vi "Variant to array strings.vi"(5 "cluster":T2(array[cluster]), 6 "Array index":string, 8 "Error out":errorcluster, 9 "Path":string, 10 "Params":T3, 11 "Variant":variant) -> (0 "Error out":errorcluster, 3 "output array":T2(array[cluster]))   [LabVIEW 2021, in "Tree.lvlib" / "Tree.lvclass"]
uses:
  Tree.lvclass
  <vilib>/Utility/Data Type/Type Definitions/Data Type.ctl
  <vilib>/Utility/Data Type/NI_Data Type.lvlib
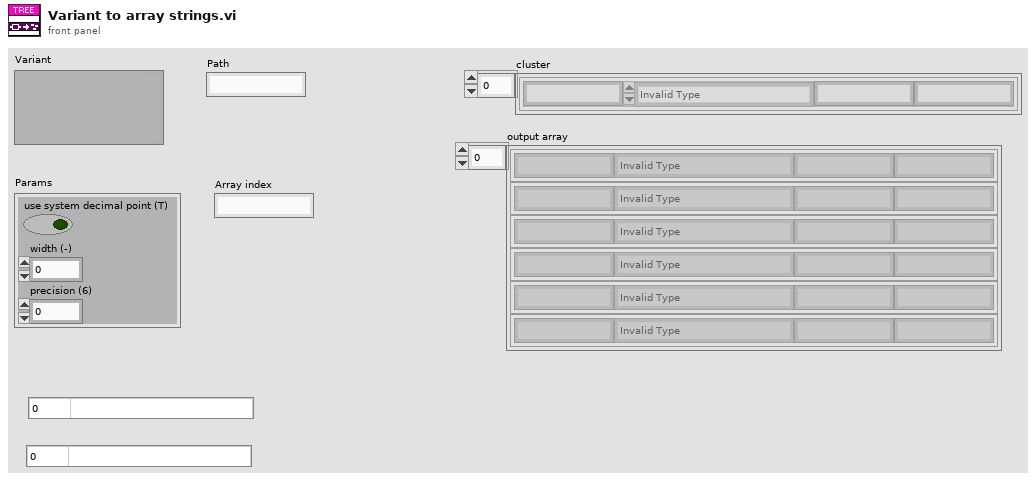
[diagram p1: front panel]
types:
  T1 = typedef "NI_Data Type.lvlib/Data Type.ctl" = enum8{"Invalid Type", "Void", "I8", "I16", "I32", "I64", "U8", "U16", "U32", "U64", "Single Float", "Double Float", "Extended Float", "Single Complex", "Double Complex", "Extended Complex", "Enum U8", "Enum U16", "Enum U32", "Enum U64", "Single Float With Unit", "Double Float With Unit", "Extended Float With Unit", "Single Complex with Unit", "Double Complex with Unit", "Extended Complex with Unit", "Boolean", "String", "Path", "Picture", "Tag", "Array", "Cluster", "Variant", "LV Variant", "Waveform", "Timestamp", "Digital Waveform", "Digital Data", "ExpressData", "Refnum", "External Data", "VI", "Poly VI", "LabVIEW Class Instance", "Fixed Point", "Set Collection", "Map Collection"}
  T2 = cluster{"Path":string, "Type":T1, "Label":string, "Value":string}[]
  T3 = cluster{"use system decimal point (T)":bool, "width (-)":i16, "precision (6)":i16}
  T4 = cluster{"Path":string, "type":T1, string, string}
  T5 = cluster{"Path":string, "type":T1, "Label":string, "Value":string}[]
  T6 = cluster{"Path":string, "type":T1, string, "Name":string}
  T7 = cluster{"Path":string, "type":T1, "Label":string, "Name":string}[]
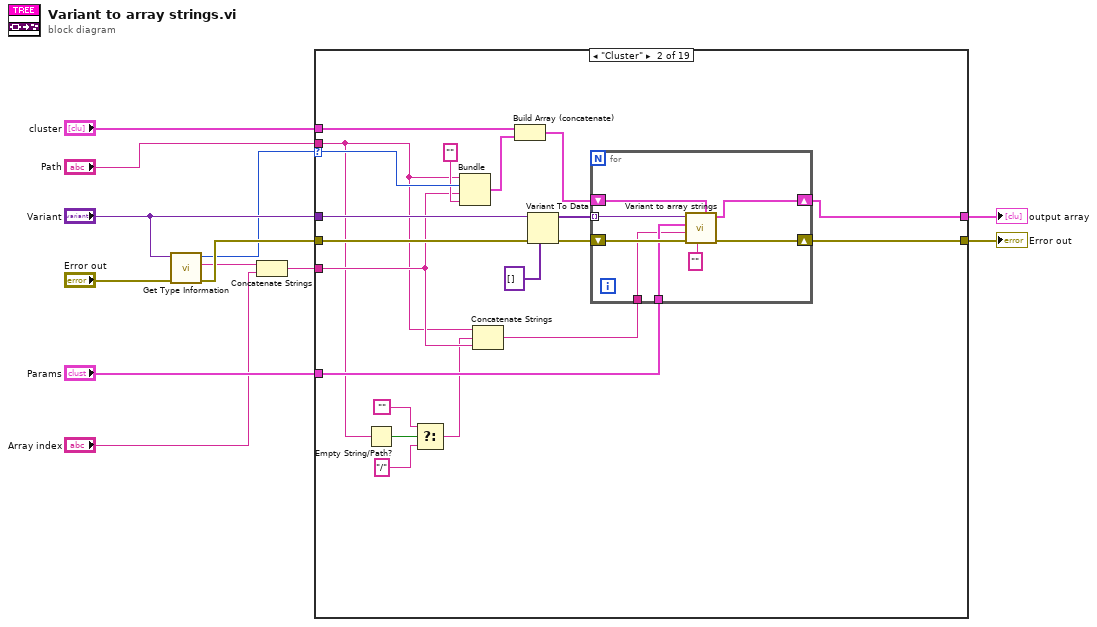
[diagram p0: block diagram]
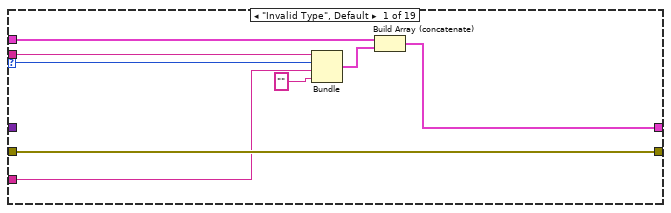
[diagram p2: hidden frame]
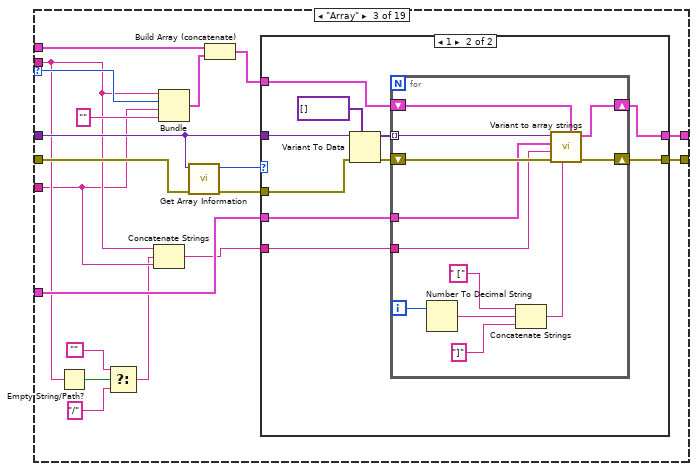
[diagram p3: hidden frame]
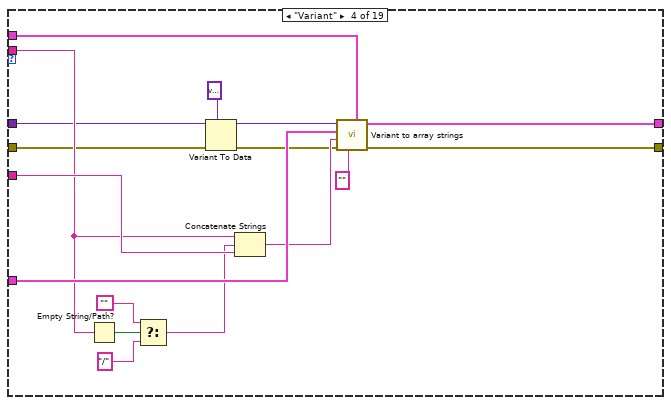
[diagram p5: hidden frame]
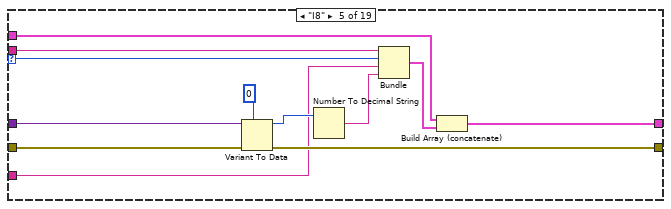
[diagram p6: hidden frame]
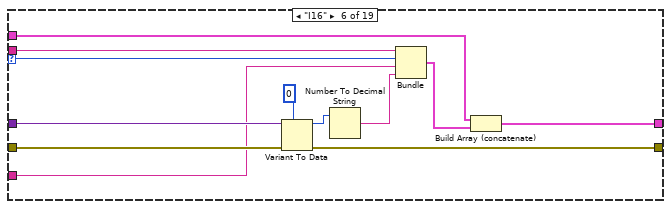
[diagram p7: hidden frame]
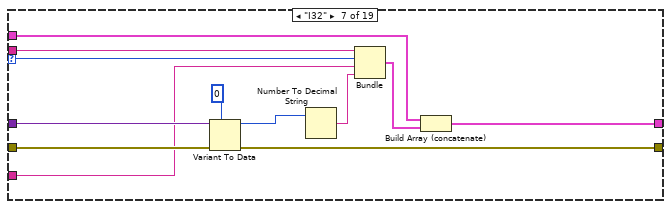
[diagram p8: hidden frame]
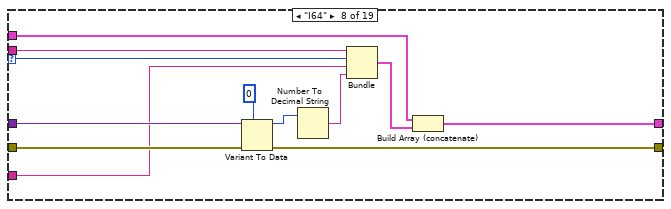
[diagram p9: hidden frame]
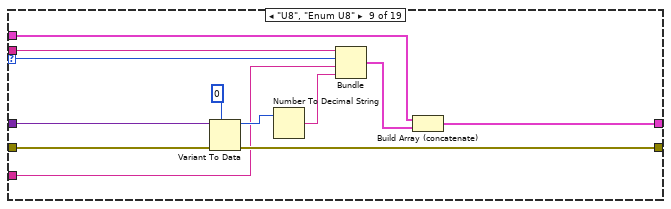
[diagram p10: hidden frame]
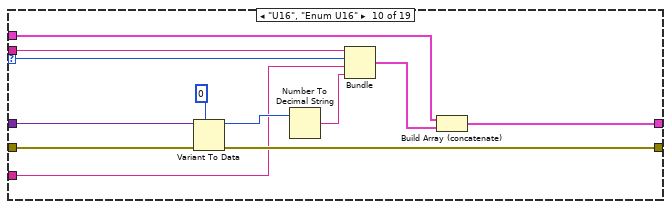
[diagram p11: hidden frame]
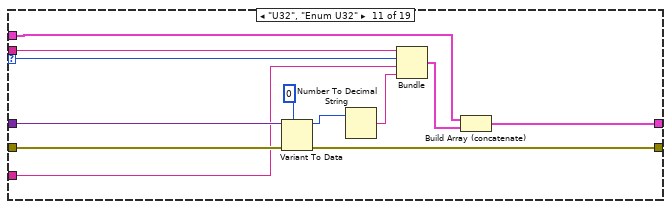
[diagram p12: hidden frame]
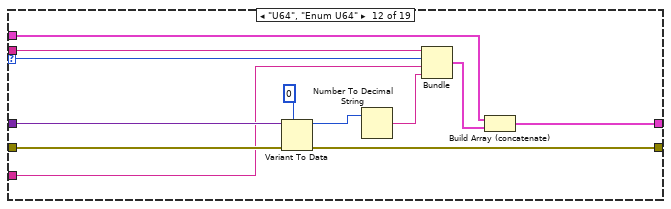
[diagram p13: hidden frame]
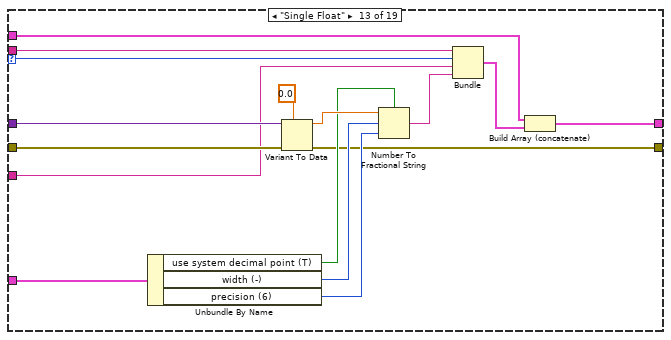
[diagram p14: hidden frame]
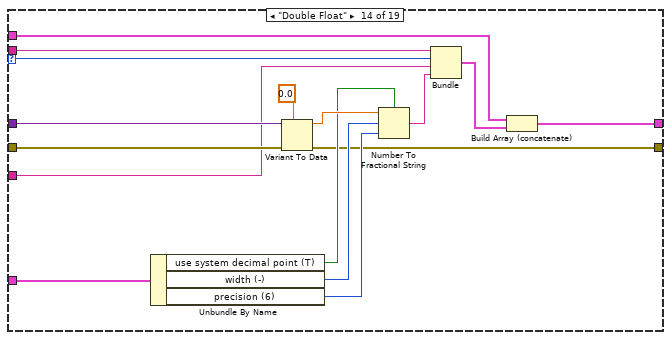
[diagram p15: hidden frame]
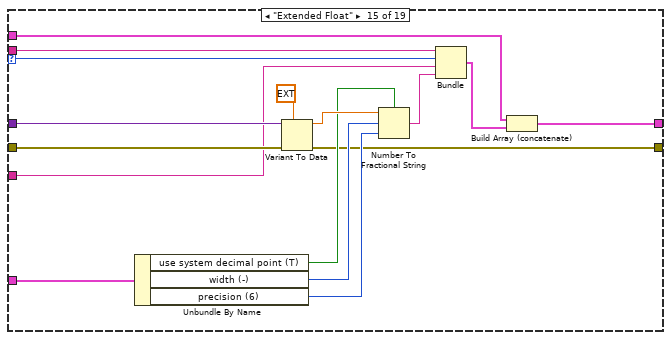
[diagram p16: hidden frame]
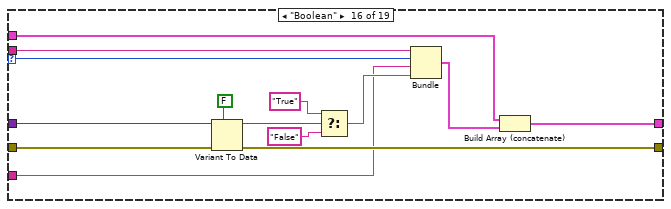
[diagram p17: hidden frame]
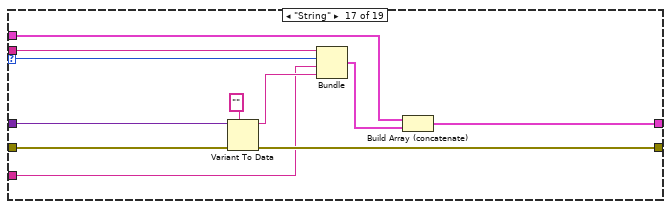
[diagram p18: hidden frame]
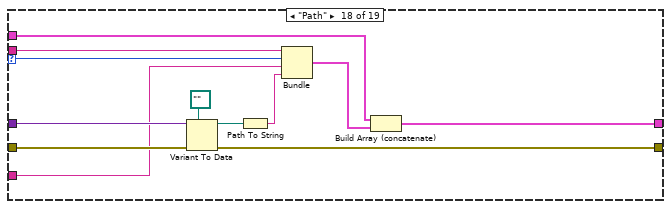
[diagram p19: hidden frame]
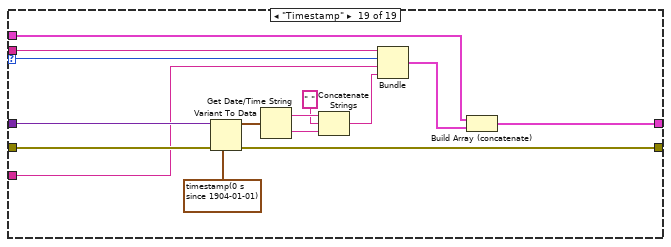
[diagram p20: hidden frame]
diagram:
  n1 = call <vilib>:"Get Type Information.vi"("error in (no error)"="Error out", "variant"="Variant") -> ("error out"=w11:errorcluster, "name"=w7:string, "type"=w9:T1)  [unwired: 5 in, 2 out]
  n2 = Concatenate Strings(w7, "Array index") -> (w2:string)
  n3 = case shown="\"Cluster\"" w9 {
    selector: w9 -> [w19 w36 w59 _ w114 w126 w138 w150 w162 w174 w186 w198 w205 w226 w242 w258 w272 w281 w295]
    tunnel: "Variant" -> [_ w33 w64 w97 w120 w132 w144 w156 w168 w180 w192 w204 w220 w236 w252 w266 w277 w289 w304]
    tunnel: w11 -> [w20 w31 w62 w94 w116 w128 w140 w152 w164 w176 w188 w200 w212 w228 w244 w264 w276 w288 w303]
    tunnel: [w20 w40 w65 w108 w115 w127 w139 w151 w163 w175 w187 w199 w211 w227 w243 w263 w275 w287 w302] -> w8
    tunnel: w2 -> [w13 w26 w50 w103 w109 w121 w133 w145 w157 w169 w181 w193 w206 w221 w237 w253 w267 w278 w290]
    tunnel: [w16 w38 w66 w106 w117 w129 w141 w153 w165 w177 w189 w201 w218 w234 w250 w260 w274 w286 w301] -> w5
    tunnel: "Params" -> [_ w39 w67 w107 _ _ _ _ _ _ _ _ w216 w232 w248 _ _ _ _]
    tunnel: "cluster" -> [w15 w37 w60 w105 w111 w123 w135 w147 w159 w171 w183 w195 w208 w223 w239 w255 w270 w280 w292]
    tunnel: "Path" -> [w14 w25 w51 w99 w110 w122 w134 w146 w158 w170 w182 w194 w207 w222 w238 w254 w268 w279 w291]
    frame "Invalid Type", Default {
      n4 = Bundle("Path"=w14, "type"=w19, w13, "") -> (w17:T4)  [unwired: 1 in]
      n5 = Build Array (concatenate)(w15, w17) -> (w16:T5)
    }
    frame "Cluster" {
      n6 = Empty String/Path?(string/path=w25) -> (empty?=w24:bool)
      n7 = Select(t="", s=w24, f="/" ("string")) -> (s? t:f=w21:string)
      n8 = Bundle("Path"=w25, "type"=w36, w26, "") -> (w27:T4)  [unwired: 1 in]
      n9 = Concatenate Strings(w25, w21, w26) -> (w35:string)
      n10 = Build Array (concatenate)(w37, w27) -> (w28:T5)
      n11 = Variant To Data(error in=w31, type=variant[] [], Variant=w33) -> (data=w29:variant[], error out=w30:errorcluster)
      n12 = for {
        shift-right: [w47] -> w40
        shift-left: w30 -> [w48]
        tunnel: w29 -> [w46] mode=indexing
        tunnel: w39 -> [w45]
        shift-right: [w42] -> w38
        shift-left: w28 -> [w44]
        tunnel: w35 -> [w43]
        n13 = call "Variant to array strings.vi"("cluster"=w44, "Array index"="", "Error out"=w48, "Path"=w43, "Params"=w45, "Variant"=w46) -> ("Error out"=w47:errorcluster, "output array"=w42:T2)  [unwired: 4 in]
      }
    }
    frame "Array" {
      n14 = Empty String/Path?(string/path=w51) -> (empty?=w54:bool)
      n15 = Select(t="", s=w54, f="/" ("string")) -> (s? t:f=w49:string)
      n16 = Concatenate Strings(w51, w49, w50) -> (w58:string)
      n17 = Bundle("Path"=w51, "type"=w59, w50, "") -> (w55:T4)  [unwired: 1 in]
      n18 = call <vilib>:"Get Array Information.vi"("error in (no error)"=w62, "variant"=w64) -> ("error out"=w61:errorcluster, "number of dimensions"=w63:i32)  [unwired: 6 in, 2 out]
      n19 = Build Array (concatenate)(w60, w55) -> (w56:T5)
      n20 = case shown="1" w63 {
        tunnel: w67 -> [_ w79]
        tunnel: [w68 w78] -> w66
        tunnel: [w69 w77] -> w65
        tunnel: w64 -> [_ w74]
        tunnel: w61 -> [w69 w73]
        tunnel: w56 -> [w68 w71]
        tunnel: w58 -> [_ w70]
        frame 0, Default {
        }
        frame 1 {
          n21 = Variant To Data(error in=w73, type=variant[] [], Variant=w74) -> (data=w75:variant[], error out=w72:errorcluster)
          n22 = for {
            tunnel: w75 -> [w91] mode=indexing
            shift-right: [w89] -> w77
            shift-left: w72 -> [w90]
            tunnel: w79 -> [w88]
            shift-right: [w87] -> w78
            shift-left: w71 -> [w86]
            tunnel: w70 -> [w85]
            i -> [w84]
            n23 = Number To Decimal String(number=w84) -> (decimal integer string=w83:string)  [unwired: 1 in]
            n24 = Concatenate Strings(" [" ("string"), w83, "]" ("string")) -> (w80:string)
            n25 = call "Variant to array strings.vi"("cluster"=w86, "Array index"=w80, "Error out"=w90, "Path"=w85, "Params"=w88, "Variant"=w91) -> ("Error out"=w89:errorcluster, "output array"=w87:T2)  [unwired: 4 in]
          }
        }
      }
    }
    frame "Variant" {
      n26 = Empty String/Path?(string/path=w99) -> (empty?=w102:bool)
      n27 = Select(t="", s=w102, f="/" ("string")) -> (s? t:f=w98:string)
      n28 = Variant To Data(error in=w94, type=variant, Variant=w97) -> (data=w95:variant, error out=w93:errorcluster)
      n29 = Concatenate Strings(w99, w98, w103) -> (w104:string)
      n30 = call "Variant to array strings.vi"("cluster"=w105, "Array index"="", "Error out"=w93, "Path"=w104, "Params"=w107, "Variant"=w95) -> ("Error out"=w108:errorcluster, "output array"=w106:T2)  [unwired: 4 in]
    }
    frame "I8" {
      n31 = Variant To Data(error in=w116, type=i8 0, Variant=w120) -> (data=w118:i8, error out=w115:errorcluster)
      n32 = Number To Decimal String(number=w118) -> (decimal integer string=w113:string)  [unwired: 1 in]
      n33 = Bundle("Path"=w110, "type"=w114, w109, w113) -> (w112:T4)  [unwired: 1 in]
      n34 = Build Array (concatenate)(w111, w112) -> (w117:T5)
    }
    frame "I16" {
      n35 = Variant To Data(error in=w128, type=i16 0, Variant=w132) -> (data=w130:i16, error out=w127:errorcluster)
      n36 = Number To Decimal String(number=w130) -> (decimal integer string=w125:string)  [unwired: 1 in]
      n37 = Bundle("Path"=w122, "type"=w126, w121, w125) -> (w124:T4)  [unwired: 1 in]
      n38 = Build Array (concatenate)(w123, w124) -> (w129:T5)
    }
    frame "I32" {
      n39 = Variant To Data(error in=w140, type=0, Variant=w144) -> (data=w142:i32, error out=w139:errorcluster)
      n40 = Number To Decimal String(number=w142) -> (decimal integer string=w137:string)  [unwired: 1 in]
      n41 = Bundle("Path"=w134, "type"=w138, w133, w137) -> (w136:T4)  [unwired: 1 in]
      n42 = Build Array (concatenate)(w135, w136) -> (w141:T5)
    }
    frame "I64" {
      n43 = Variant To Data(error in=w152, type=i64 0, Variant=w156) -> (data=w154:i64, error out=w151:errorcluster)
      n44 = Number To Decimal String(number=w154) -> (decimal integer string=w149:string)  [unwired: 1 in]
      n45 = Bundle("Path"=w146, "type"=w150, w145, w149) -> (w148:T4)  [unwired: 1 in]
      n46 = Build Array (concatenate)(w147, w148) -> (w153:T5)
    }
    frame "U8", "Enum U8" {
      n47 = Variant To Data(error in=w164, type=u8 0, Variant=w168) -> (data=w166:u8, error out=w163:errorcluster)
      n48 = Number To Decimal String(number=w166) -> (decimal integer string=w161:string)  [unwired: 1 in]
      n49 = Bundle("Path"=w158, "type"=w162, w157, w161) -> (w160:T4)  [unwired: 1 in]
      n50 = Build Array (concatenate)(w159, w160) -> (w165:T5)
    }
    frame "U16", "Enum U16" {
      n51 = Variant To Data(error in=w176, type=u16 0, Variant=w180) -> (data=w178:u16, error out=w175:errorcluster)
      n52 = Number To Decimal String(number=w178) -> (decimal integer string=w173:string)  [unwired: 1 in]
      n53 = Bundle("Path"=w170, "type"=w174, w169, w173) -> (w172:T4)  [unwired: 1 in]
      n54 = Build Array (concatenate)(w171, w172) -> (w177:T5)
    }
    frame "U32", "Enum U32" {
      n55 = Variant To Data(error in=w188, type=u32 0, Variant=w192) -> (data=w190:u32, error out=w187:errorcluster)
      n56 = Number To Decimal String(number=w190) -> (decimal integer string=w185:string)  [unwired: 1 in]
      n57 = Bundle("Path"=w182, "type"=w186, w181, w185) -> (w184:T4)  [unwired: 1 in]
      n58 = Build Array (concatenate)(w183, w184) -> (w189:T5)
    }
    frame "U64", "Enum U64" {
      n59 = Variant To Data(error in=w200, type=u64 0, Variant=w204) -> (data=w202:u64, error out=w199:errorcluster)
      n60 = Number To Decimal String(number=w202) -> (decimal integer string=w197:string)  [unwired: 1 in]
      n61 = Bundle("Path"=w194, "type"=w198, w193, w197) -> (w196:T4)  [unwired: 1 in]
      n62 = Build Array (concatenate)(w195, w196) -> (w201:T5)
    }
    frame "Single Float" {
      n63 = Unbundle By Name(w216) -> ("use system decimal point (T)"=w215:bool, "width (-)"=w214:i16, "precision (6)"=w213:i16)
      n64 = Variant To Data(error in=w212, type=sgl 0.0, Variant=w220) -> (data=w217:sgl, error out=w211:errorcluster)
      n65 = Number To Fractional String(use system decimal point (T)=w215, number=w217, width (-)=w214, precision (6)=w213) -> (F-format string=w210:string)
      n66 = Bundle("Path"=w207, "type"=w205, w206, w210) -> (w209:T4)  [unwired: 1 in]
      n67 = Build Array (concatenate)(w208, w209) -> (w218:T5)
    }
    frame "Double Float" {
      n68 = Unbundle By Name(w232) -> ("use system decimal point (T)"=w231:bool, "width (-)"=w230:i16, "precision (6)"=w229:i16)
      n69 = Variant To Data(error in=w228, type=0.0, Variant=w236) -> (data=w233:dbl, error out=w227:errorcluster)
      n70 = Number To Fractional String(use system decimal point (T)=w231, number=w233, width (-)=w230, precision (6)=w229) -> (F-format string=w225:string)
      n71 = Bundle("Path"=w222, "type"=w226, w221, w225) -> (w224:T4)  [unwired: 1 in]
      n72 = Build Array (concatenate)(w223, w224) -> (w234:T5)
    }
    frame "Extended Float" {
      n73 = Unbundle By Name(w248) -> ("use system decimal point (T)"=w247:bool, "width (-)"=w246:i16, "precision (6)"=w245:i16)
      n74 = Variant To Data(error in=w244, type=ext 0.0, Variant=w252) -> (data=w249:ext, error out=w243:errorcluster)
      n75 = Number To Fractional String(use system decimal point (T)=w247, number=w249, width (-)=w246, precision (6)=w245) -> (F-format string=w241:string)
      n76 = Bundle("Path"=w238, "type"=w242, w237, w241) -> (w240:T4)  [unwired: 1 in]
      n77 = Build Array (concatenate)(w239, w240) -> (w250:T5)
    }
    frame "Boolean" {
      n78 = Variant To Data(error in=w264, type=FALSE, Variant=w266) -> (data=w262:bool, error out=w263:errorcluster)
      n79 = Select(t="True" ("Name"), s=w262, f="False" ("Name")) -> (s? t:f=w257:string)
      n80 = Bundle("Path"=w254, "type"=w258, w253, "Name"=w257) -> (w256:T6)  [unwired: 1 in]
      n81 = Build Array (concatenate)(w255, w256) -> (w260:T7)
    }
    frame "String" {
      n82 = Variant To Data(error in=w276, type="" ("Name"), Variant=w277) -> (data=w269:string, error out=w275:errorcluster)
      n83 = Bundle("Path"=w268, "type"=w272, w267, "Name"=w269) -> (w271:T6)  [unwired: 1 in]
      n84 = Build Array (concatenate)(w270, w271) -> (w274:T7)
    }
    frame "Path" {
      n85 = Variant To Data(error in=w288, type=path "" ("file path (use dialog)"), Variant=w289) -> (data=w285:path, error out=w287:errorcluster)
      n86 = Path To String(path=w285) -> (string=w283:string)
      n87 = Bundle("Path"=w279, "type"=w281, w278, w283) -> (w282:T4)  [unwired: 1 in]
      n88 = Build Array (concatenate)(w280, w282) -> (w286:T5)
    }
    frame "Timestamp" {
      n89 = Variant To Data(error in=w303, type=timestamp(0 s since 1904-01-01) ("current time"), Variant=w304) -> (data=w299:timestamp, error out=w302:errorcluster)
      n90 = Get Date/Time String(seconds (now)=w299) -> (date string=w298:string, time string=w297:string)  [unwired: 2 in]
      n91 = Concatenate Strings(w298, " " ("date string"), w297) -> (w294:string)
      n92 = Bundle("Path"=w291, "type"=w295, w290, w294) -> (w293:T4)  [unwired: 1 in]
      n93 = Build Array (concatenate)(w292, w293) -> (w301:T5)
    }
  }
  "output array" <- w5
  "Error out" <- w8
